vi "CRYWave Resolve Convert.vi"(8 "Y Resolution":u8=1 caption="Absolute Comparison Precision", 10 "X Resolution":u8=1 caption="Absolute Comparison Precision" format="%01.0f", 11 "Data Wave":T1={"Waveform"={"X0"=0.0, "dX"=0.0, "Y"=[]}, "X data"=1, "Y data"=1, "Y axis"=1, "X unit"="s", "Y unit"="V", "Y dB ref"=1.0, "display Y"=TRUE, "display X"=TRUE, "Overload?"=FALSE, "Test Info"="", "Step No."=0, "Name"="", "protected"=FALSE, "Sqc history"=[], "Signal Channel ID"=0, "Plot Settings"={"Color"=0, "Interpolation"=0, "Point Style"=0, "Line Style"=0, "Point Color"=0, "Line Width"=0, "Bar Plot Style"=0, "Fill To"=0}, "AutoProtect"=FALSE} {"Y dB ref" format="%.1f"; "Y axis" items=["Log", "Lin"]; "Y data" items=["dB", "Lin"]; "X data" items=["dB", "Lin"]}) -> (3 "Curve Out":cluster{dbl, dbl}[](array[cluster]))   [LabVIEW 2013]
uses:
  Typedef Control/CRYWaveform Cluster.ctl
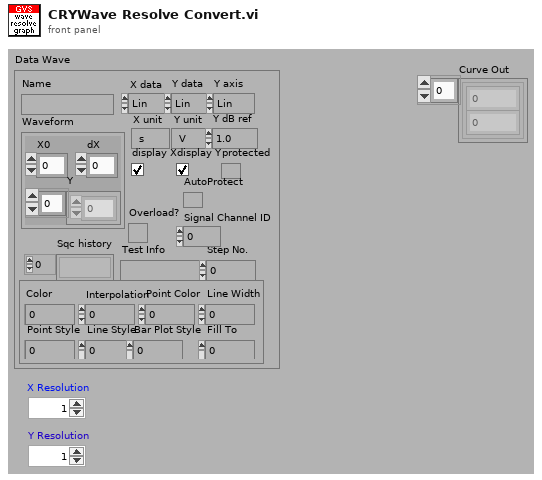
[diagram p1: front panel]
types:
  T1 = typedef "CRYWaveform Cluster.ctl" = cluster{"Waveform":cluster{"X0":dbl, "dX":dbl, "Y":sgl[]}, "X data":u16, "Y data":u16, "Y axis":u16, "X unit":string, "Y unit":string, "Y dB ref":dbl, "display Y":bool, "display X":bool, "Overload?":bool, "Test Info":string, "Step No.":i32, "Name":string, "protected":bool, "Sqc history":string[], "Signal Channel ID":i32, "Plot Settings":cluster{"Color":u32, "Interpolation":u8, "Point Style":u8, "Line Style":u8, "Point Color":u32, "Line Width":u8, "Bar Plot Style":u8, "Fill To":i16}, "AutoProtect":bool}
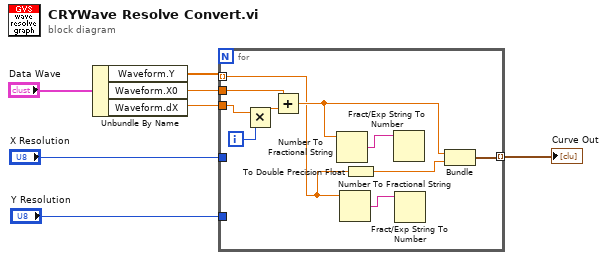
[diagram p0: block diagram]
diagram:
  n1 = Unbundle By Name("Data Wave") -> ("Waveform.Y"=w6:sgl[], "Waveform.X0"=w5:dbl, "Waveform.dX"=w4:dbl)
  n2 = for {
    tunnel: w4 -> [w17]
    tunnel: w5 -> [w15]
    tunnel: w6 -> [w9] mode=indexing
    tunnel: "X Resolution" -> [_]
    tunnel: "Y Resolution" -> [_]
    tunnel: [w11] -> w1 mode=indexing
    i -> [w14]
    n3 = Multiply(x=w17, y=w14) -> (x*y=w16:dbl)
    n4 = Add(x=w15, y=w16) -> (x+y=w10:dbl)
    n5 = Number To Fractional String(number=w10) -> (F-format string=w13:string)  [unwired: 3 in]
    n6 = Number To Fractional String(number=w9) -> (F-format string=w12:string)  [unwired: 3 in]
    n7 = To Double Precision Float(number=w9) -> (double precision float=w8:dbl)
    n8 = Fract/Exp String To Number(string=w13) -> ()  [unwired: 3 in, 2 out]
    n9 = Fract/Exp String To Number(string=w12) -> ()  [unwired: 3 in, 2 out]
    n10 = Bundle(w10, w8) -> (w11:cluster{dbl, dbl})  [unwired: 1 in]
  }
  "Curve Out" <- w1
